vi "Variant2String.vi"(8 "error in":errorcluster, 11 "variant array":variant[](array[variant])) -> (0 "error out":errorcluster, 3 "string array":string[](array[string]))   [LabVIEW 2011]
panel:
  out "Array 2":u32[](array[numeric])
  out "Array":string[](array[string])
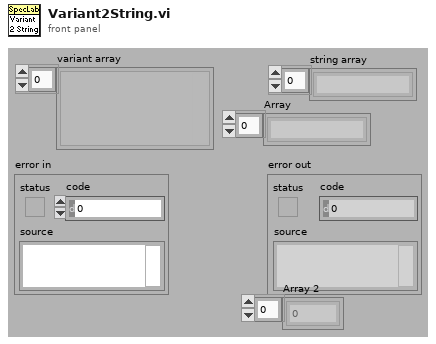
[diagram p1: front panel]
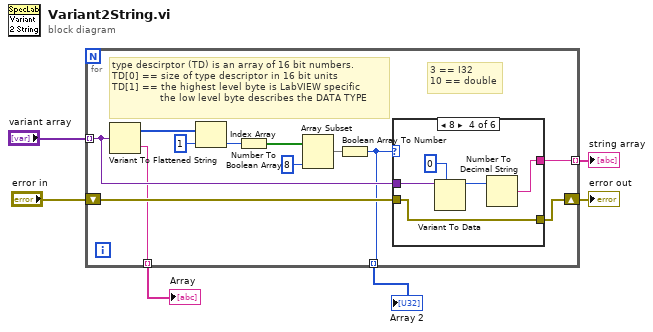
[diagram p0: block diagram]
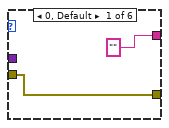
[diagram p2: hidden frame]
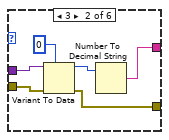
[diagram p3: hidden frame]
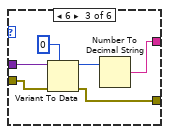
[diagram p4: hidden frame]
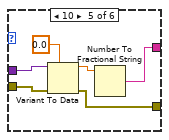
[diagram p5: hidden frame]
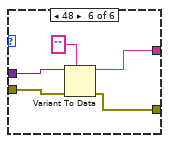
[diagram p6: hidden frame]
diagram:
  n1 = for {
    tunnel: [w12] -> w5 mode=indexing
    tunnel: "variant array" -> [w9] mode=indexing
    shift-right: [w10] -> w3
    shift-left: "error in" -> [w11]
    tunnel: [w8] -> w2 mode=indexing
    tunnel: [w7] -> w1 mode=indexing
    # "3 == I32\n10 == double"
    # "type descirptor (TD) is an array of 16 bit numbers.\nTD[0] == size of type descriptor in 16 bit units\nTD[1] == the highest level byte is LabVIEW specific\n                the low level byte describes the DATA TYPE"
    n2 = Variant To Flattened String(Variant=w9) -> (data string=w8:string, 1:w18:i16[])
    n3 = Index Array(array=w18, index=1) -> (element=w16:i16)
    n4 = Number To Boolean Array(number=w16) -> (Boolean array=w15:bool[])
    n5 = Array Subset(array=w15, length=8) -> (w13:bool[])  [unwired: 1 in]
    n6 = Boolean Array To Number(Boolean array=w13) -> (number=w7:u32)
    n7 = case shown="8" w7 {
      tunnel: ["" w24 w27 w33 w41 w47] -> w12
      tunnel: w11 -> [w19 w23 w29 w34 w40 w46]
      tunnel: [w19 w22 w28 w34 w39 w45] -> w10
      tunnel: w9 -> [_ w21 w30 w35 w38 w44]
      frame 0, Default {
      }
      frame 3 {
        n8 = Variant To Data(error in=w23, type=0 ("y"), Variant=w21) -> (data=w25:i32, error out=w22:errorcluster)
        n9 = Number To Decimal String(number=w25) -> (decimal integer string=w24:string)  [unwired: 1 in]
      }
      frame 6 {
        n10 = Variant To Data(error in=w29, type=u16 0 ("y"), Variant=w30) -> (data=w31:u16, error out=w28:errorcluster)
        n11 = Number To Decimal String(number=w31) -> (decimal integer string=w27:string)  [unwired: 1 in]
      }
      frame 8 {
        n12 = Variant To Data(type=u64 0 ("y"), Variant=w35) -> (data=w36:u64)  [unwired: 1 in, 1 out]
        n13 = Number To Decimal String(number=w36) -> (decimal integer string=w33:string)  [unwired: 1 in]
      }
      frame 10 {
        n14 = Variant To Data(error in=w40, type=0.0 ("y"), Variant=w38) -> (data=w42:dbl, error out=w39:errorcluster)
        n15 = Number To Fractional String(number=w42) -> (F-format string=w41:string)  [unwired: 3 in]
      }
      frame 48 {
        n16 = Variant To Data(error in=w46, type="", Variant=w44) -> (data=w47:string, error out=w45:errorcluster)
      }
    }
  }
  "string array" <- w5
  "error out" <- w3
  "Array" <- w2
  "Array 2" <- w1
